vi "GV-GetLegendRange.vi"(8 "error in (no error)":errorcluster, 9 "Coords":T1, 11 "Gviewer in":refnum<class "Gviewer.lvclass">) -> (0 "error out":errorcluster, 1 "Where?":enum16{"Scroll over Plot", "Scroll over Legend"}(ring), 3 "Gviewer out":refnum<class "Gviewer.lvclass">)   [LabVIEW 2020, in "Sgraph_lib_V1.lvlib" / "Gviewer.lvclass"]
doc: "Andre Koelewijn, 25 April 2021\n\nCheck if the mouse is hovering over the Legend section or not"
uses:
  Gviewer.lvclass
  <vilib>/Utility/miscctls.llb/LVPoint32TypeDef.ctl
  Gviewer.lvclass/Gviewer.ctl
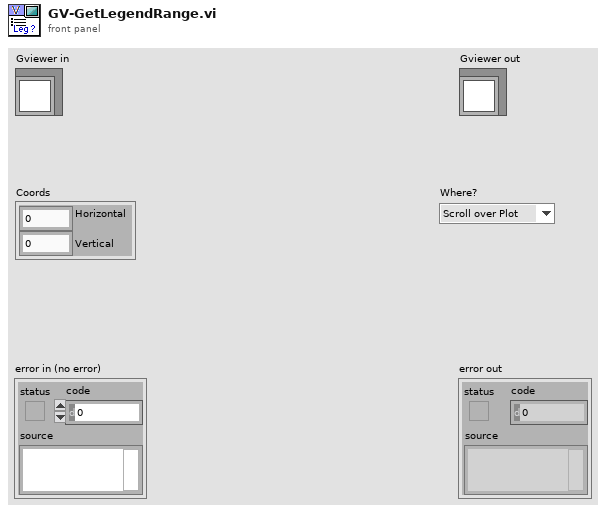
[diagram p1: front panel]
types:
  T1 = typedef "LVPoint32TypeDef.ctl" = cluster{"Horizontal":i32, "Vertical":i32}
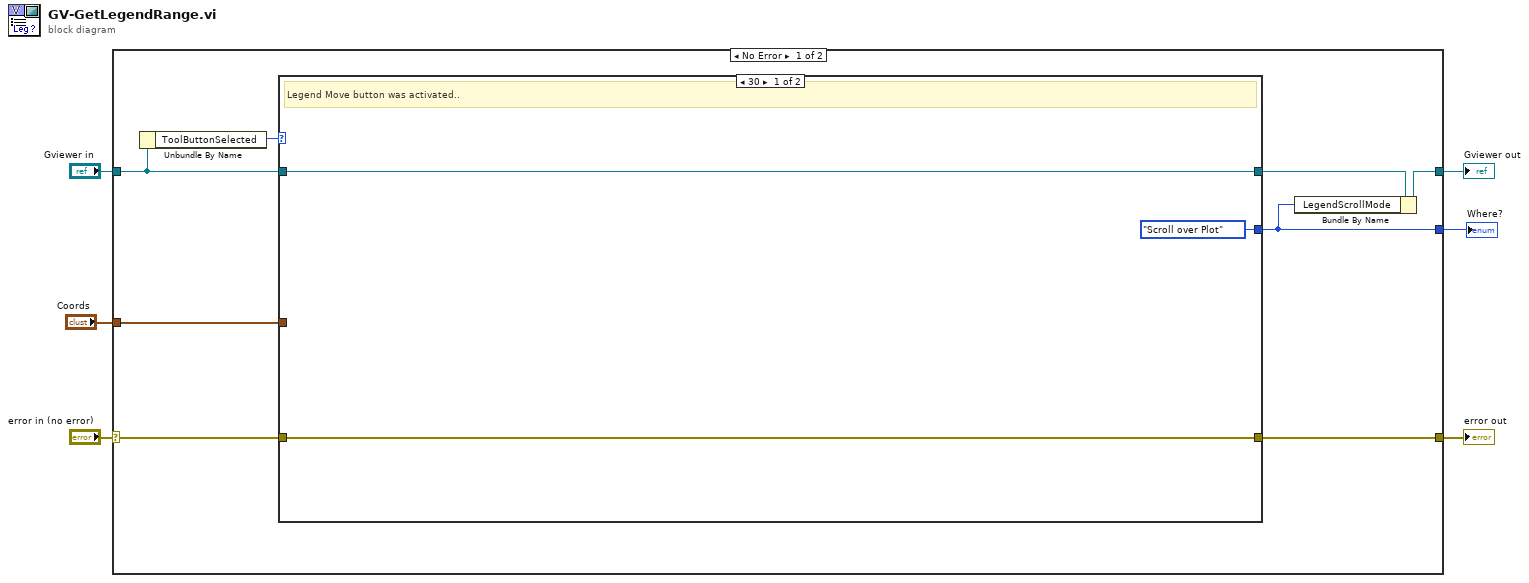
[diagram p0: block diagram]
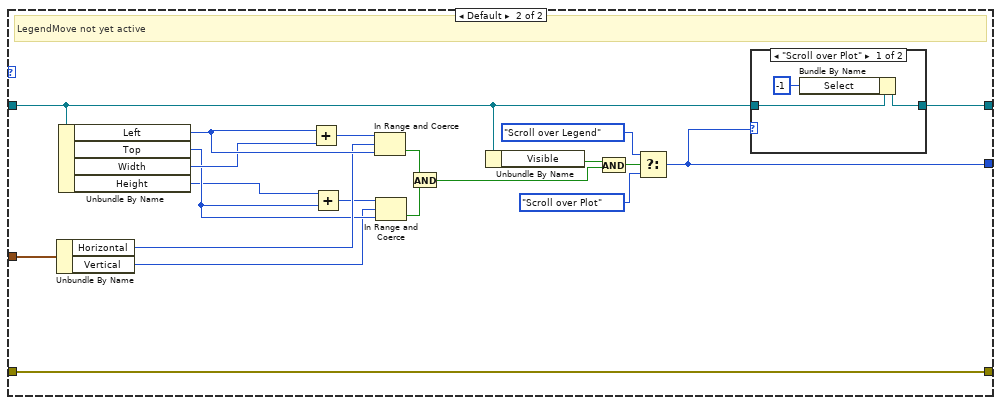
[diagram p2: hidden frame]
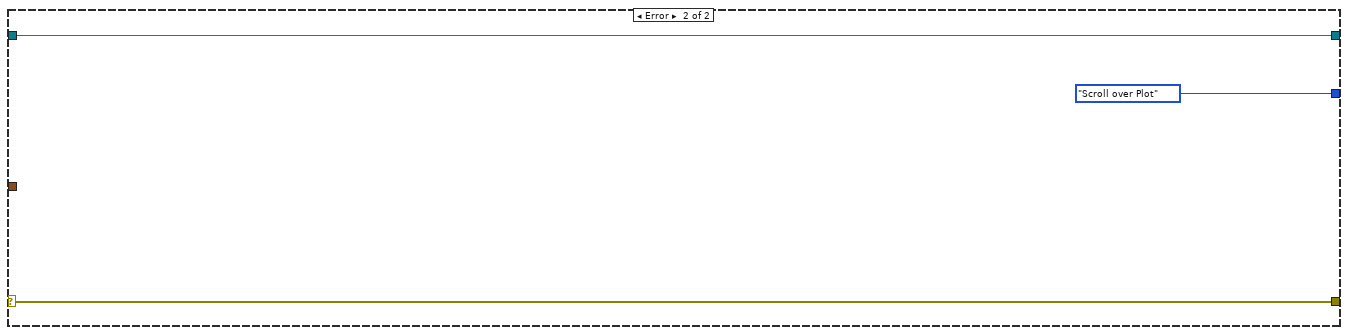
[diagram p4: hidden frame]
diagram:
  n1 = case shown="No Error" "error in (no error)" {
    selector: "error in (no error)" -> [w11 w44]
    tunnel: [w10 w44] -> w5
    tunnel: [w7 w43] -> w3
    tunnel: "Gviewer in" -> [w13 w43]
    tunnel: "Coords" -> [w14 _]
    tunnel: [w9 enum16{"Scroll over Plot", "Scroll over Legend"}."Scroll over Plot" ("Where?")] -> w1
    frame No Error {
      n2 = Unbundle By Name(w13) -> ("ToolButtonSelected"=w12:i32)
      n3 = case shown="30" w12 {
        tunnel: w14 -> [_ w37]
        tunnel: [enum16{"Scroll over Plot", "Scroll over Legend"}."Scroll over Plot" ("Where?") w21] -> w9
        tunnel: [w17 w20] -> w8
        tunnel: w13 -> [w17 w19]
        tunnel: w11 -> [w16 w18]
        tunnel: [w16 w18] -> w10
        frame 30 {
          # "Legend Move button was activated.."
        }
        frame Default {
          # "LegendMove not yet active"
          n4 = Unbundle By Name(w37) -> ("Horizontal"=w33:i32, "Vertical"=w29:i32)
          n5 = Unbundle By Name(w19) -> ("Left"=w36:i32, "Top"=w32:i32, "Width"=w35:u32, "Height"=w31:u32)
          n6 = Add(x=w36, y=w35) -> (x+y=w34:u32)
          n7 = Add(x=w31, y=w32) -> (x+y=w30:u32)
          n8 = In Range and Coerce(upper limit=w34, x=w33, lower limit=w36) -> (In Range?=w28:bool)  [unwired: 1 out]
          n9 = In Range and Coerce(upper limit=w30, x=w29, lower limit=w32) -> (In Range?=w27:bool)  [unwired: 1 out]
          n10 = And(x=w28, y=w27) -> (x .and. y?=w25:bool)
          n11 = Unbundle By Name(w19) -> ("Visible"=w26:bool)
          n12 = And(x=w26, y=w25) -> (x .and. y?=w24:bool)
          n13 = Select(t=enum16{"Scroll over Plot", "Scroll over Legend"}."Scroll over Legend" ("Where?"), s=w24, f=enum16{"Scroll over Plot", "Scroll over Legend"}."Scroll over Plot" ("Where?")) -> (s? t:f=w21:enum16{"Scroll over Plot", "Scroll over Legend"})
          n14 = case shown="\"Scroll over Plot\"" w21 {
            tunnel: w19 -> [w40 w41]
            tunnel: [w39 w41] -> w20
            frame "Scroll over Plot" {
              n15 = Bundle By Name(cluster=w40, "Select"=-1 ("Legend.Select")) -> (w39:refnum<class "Gviewer.lvclass">)
            }
            frame "Scroll over Legend" {
            }
          }
        }
      }
      n16 = Bundle By Name(cluster=w8, "LegendScrollMode"=w9) -> (w7:refnum<class "Gviewer.lvclass">)
    }
    frame Error {
    }
  }
  "error out" <- w5
  "Gviewer out" <- w3
  "Where?" <- w1
